vi "update_#scans.vi"(8 "error in (no error)":errorcluster, 10 "# scans":i32, 11 "Detector in":refnum<class "Detector.lvclass">) -> (0 "error out":errorcluster, 3 "Detector out":refnum<class "Detector.lvclass">)   [LabVIEW 2020, in "Detector.lvclass"]
uses:
  Detector.lvclass
  Detector.lvclass/Detector.ctl
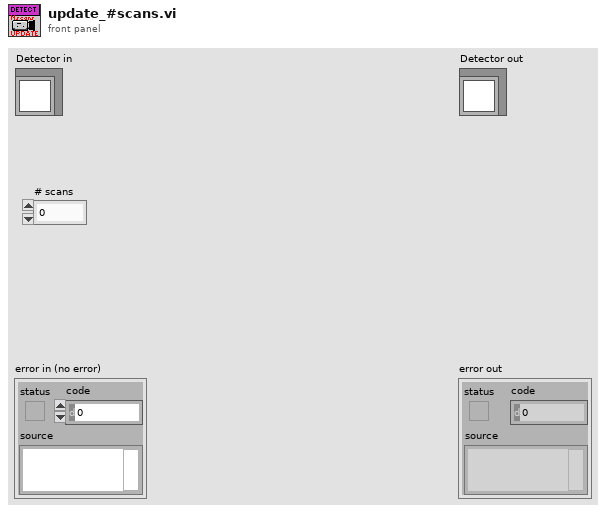
[diagram p1: front panel]
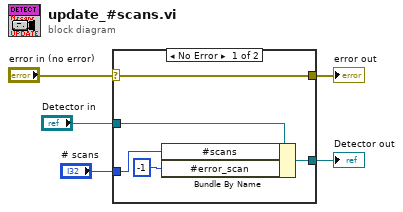
[diagram p0: block diagram]
diagram:
  n1 = case shown="No Error" "error in (no error)" {
    selector: "error in (no error)" -> [w10 w12]
    tunnel: [w10 w12] -> w4
    tunnel: [w8 w11] -> w2
    tunnel: "Detector in" -> [w9 w11]
    tunnel: "# scans" -> [w7 _]
    frame No Error {
      n2 = Bundle By Name(cluster=w9, "#scans"=w7, "#error_scan"=-1 ("error_OD.#error_scan")) -> (w8:refnum<class "Detector.lvclass">)
    }
    frame Error {
    }
  }
  "error out" <- w4
  "Detector out" <- w2
